vi "Write (append).vi"(8 "error in (no error)":errorcluster, 11 "Write (append) this text to the file":string) -> (0 "error out":errorcluster)   [LabVIEW 2018, in "text_file.lvlib"]
uses:
  text_file.lvlib
  private_data (library_variable).vi
panel:
  # "Development\ncontrols/indicators useful for development and testing, but which are not outputs of the VI"
  # "Input\nInputs to the VI"
  # "Output\nOutputs of the VI"
  # "Description\n\nBlank VI with error handling case. \n\nSummarize the use of this VI in this space."
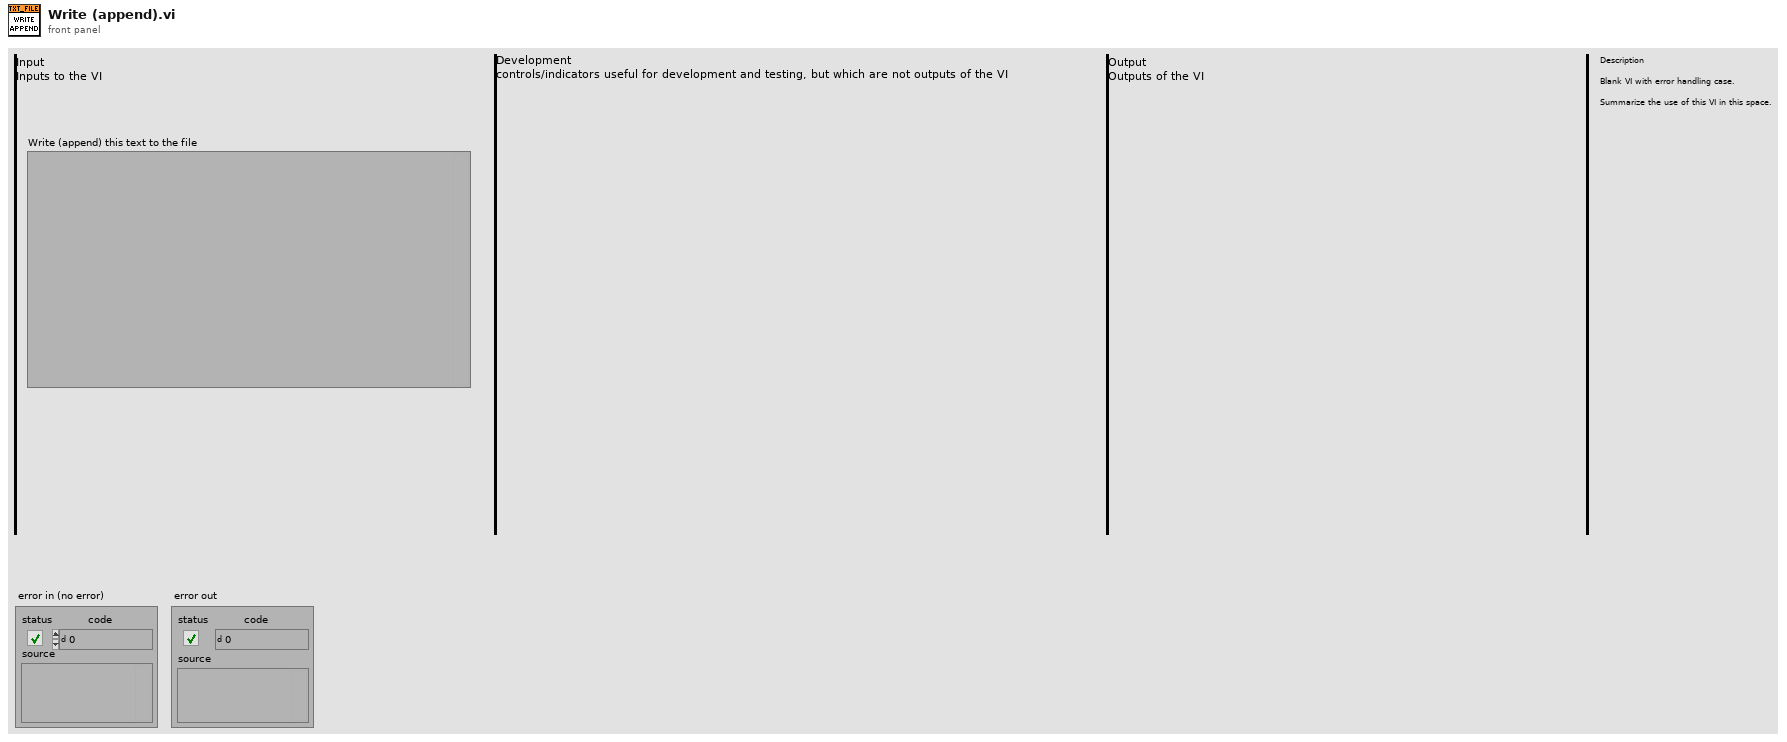
[diagram p1: front panel]
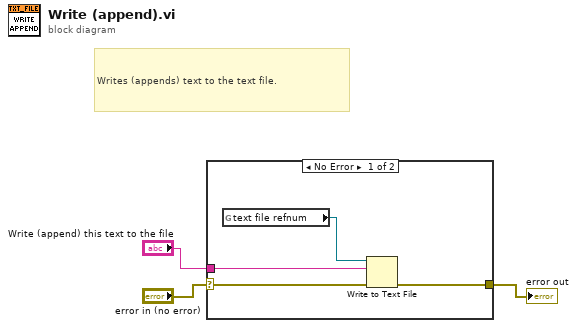
[diagram p0: block diagram]
diagram:
  # "Writes (appends) text to the text file."
  n1 = case shown="No Error" "error in (no error)" {
    selector: "error in (no error)" -> [w7 w8]
    tunnel: [w6 w8] -> w2
    tunnel: "Write (append) this text to the file" -> [w4 _]
    frame No Error {
      n2 = global read "private_data (library_variable).vi" "text file refnum"() -> (w5:refnum<file>)
      n3 = Write to Text File(file (use dialog)=w5, text=w4, error in=w7) -> (error out=w6:errorcluster)  [unwired: 1 in, 2 out]
    }
    frame Error {
    }
  }
  "error out" <- w2
